vi "Form Error Log Text.vi"(11 "Error Source Input":string) -> (3 "String to Write":string)   [LabVIEW 2015, in "Generic Module Library.lvlib" / "Template G_Module.lvlib"]
uses:
  Template G_Module.lvlib
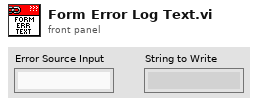
[diagram p1: front panel]
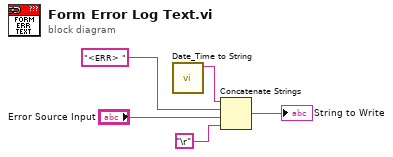
[diagram p0: block diagram]
diagram:
  n1 = call "Date_Time to String.vi"() -> ("date/time string"=w2:string)  [unwired: 11 in]
  n2 = Concatenate Strings(w2, "<ERR> " ("string"), "Error Source Input", "\r") -> (→"String to Write":string)
